vi "Set_up_controls.vi"(4 "error in":errorcluster, 5 "reference":refnum<vi>, 6 "FP refnum in":cluster{"server refnum":u32, "tag refnum":u32}, 7 "Data in":T1) -> (0 "error out":errorcluster, 1 "reference out":refnum<vi>, 2 "FP refnum out":cluster{"server refnum":u32, "tag refnum":u32}, 3 "Data out":T1)   [LabVIEW 2015, in "Steps.lvlib"]
uses:
  Steps.lvlib
  Type_Defs/Data.ctl
  Type_Defs/Diagnostics.ctl
  Type_Defs/Systems.ctl
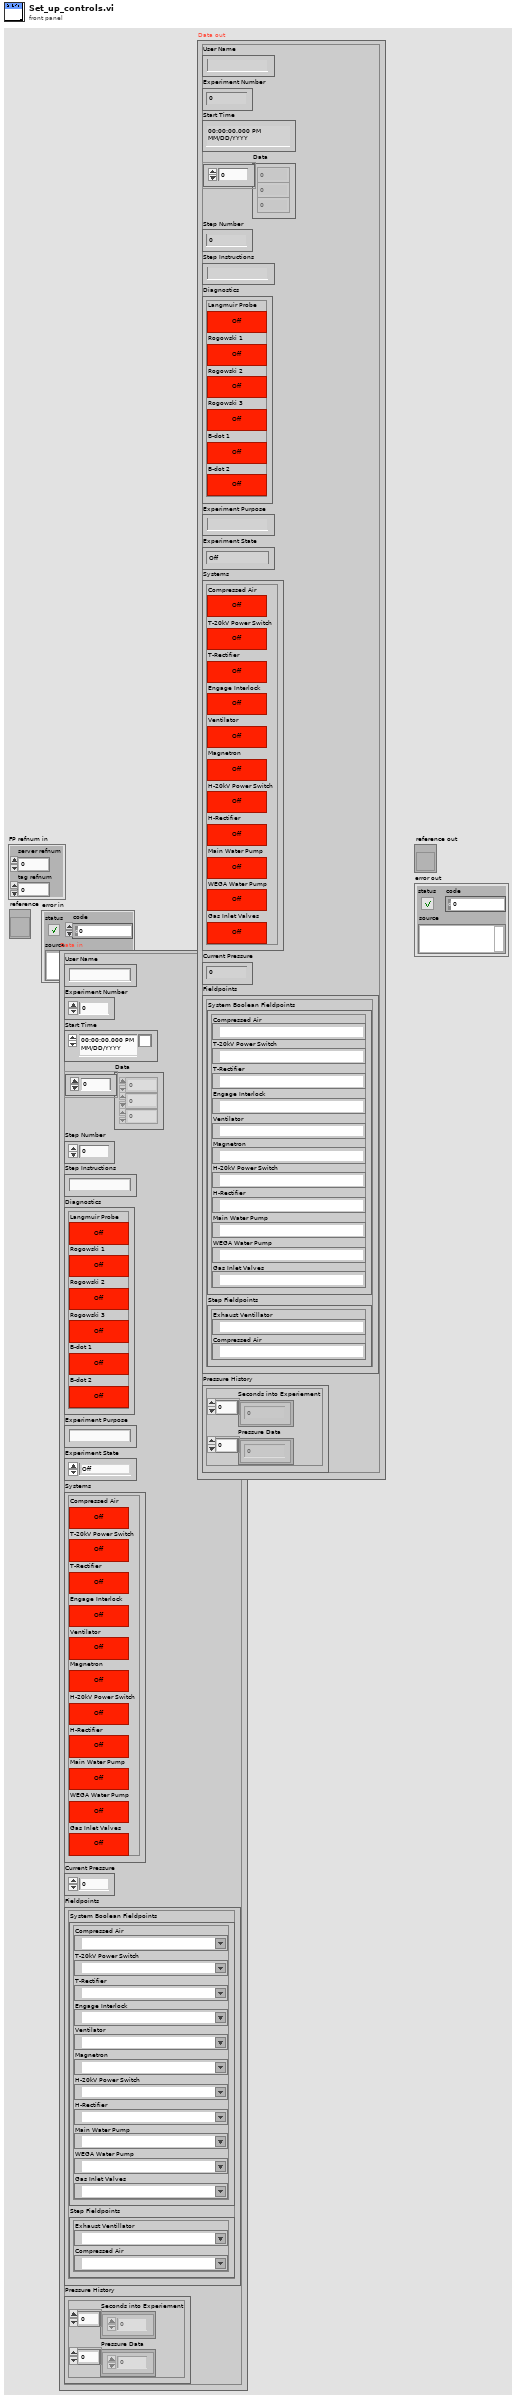
[diagram p1: front panel]
types:
  T1 = typedef "Data.ctl" = cluster{"User Name":string, "Experiment Number":i32, "Start Time":timestamp, "Data":dbl[], "Step Number":i32, "Step Instructions":string, "Diagnostics":T2, "Experiment Purpose":string, "Experiment State":enum16{"Off", "Setting Up", "Ready", "In Progress", "Shutting Down"}, "Systems":T3, "Current Pressure":dbl, "Fieldpoints":cluster{"System Boolean Fieldpoints":cluster{"Compressed Air":refnum<k21>, "T-20kV Power Switch":refnum<k21>, "T-Rectifier":refnum<k21>, "Engage Interlock":refnum<k21>, "Ventilator":refnum<k21>, "Magnetron":refnum<k21>, "H-20kV Power Switch":refnum<k21>, "H-Rectifier":refnum<k21>, "Main Water Pump":refnum<k21>, "WEGA Water Pump":refnum<k21>, "Gas Inlet Valves":refnum<k21>}, "Step Fieldpoints":cluster{"Exhaust Ventillator":refnum<k21>, "Compressed Air":refnum<k21>}}, "Pressure History":cluster{"Seconds into Experiement":i32[], "Pressure Data":dbl[]}}
  T2 = typedef "Diagnostics.ctl" = cluster{"Langmuir Probe":bool, "Rogowski 1":bool, "Rogowski 2":bool, "Rogowski 3":bool, "B-dot 1":bool, "B-dot 2":bool}
  T3 = typedef "Systems.ctl" = cluster{"Compressed Air":bool, "T-20kV Power Switch":bool, "T-Rectifier":bool, "Engage Interlock":bool, "Ventilator":bool, "Magnetron":bool, "H-20kV Power Switch":bool, "H-Rectifier":bool, "Main Water Pump":bool, "WEGA Water Pump":bool, "Gas Inlet Valves":bool}
  T4 = enum16{"Off", "Setting Up", "Ready", "In Progress", "Shutting Down"}
  T5 = enum8{"Enabled", "Disabled", "Disabled and Grayed Out"}
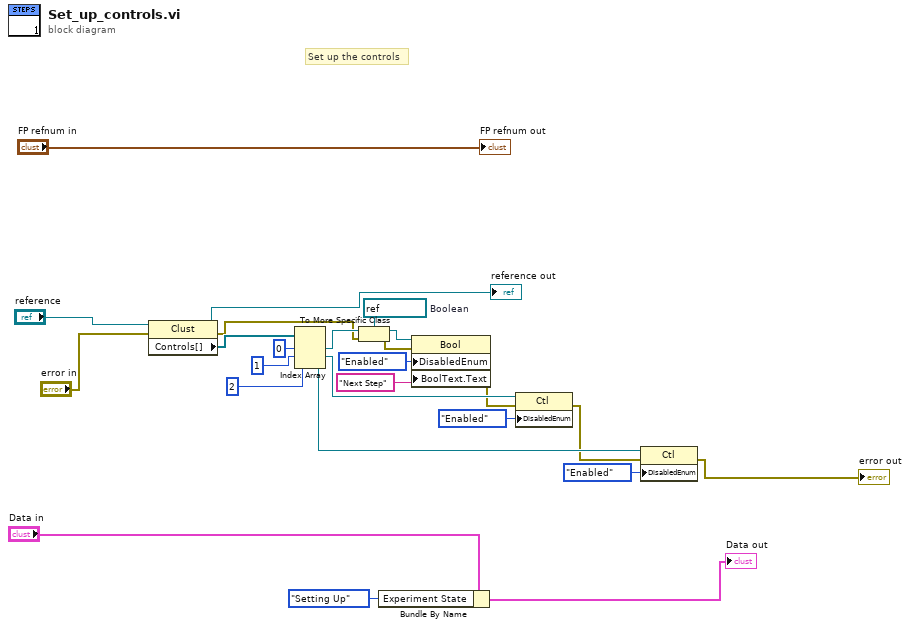
[diagram p0: block diagram]
diagram:
  w5 = refnum<vi> refnum  # Boolean
  # "Set up the controls"
  n1 = property class="Clust"(reference="reference", error in="error in") -> (reference out=→"reference out":refnum<vi>, error out=w8:errorcluster, "Controls[]"=w25:refnum<vi>[])
  n2 = Index Array(array=w25, index #1=0 ("index"), index #2=1 ("index"), index #3=2 ("index")) -> (element #1=w9:refnum<vi>, element #2=w21:refnum<vi>, element #3=w20:refnum<vi>)
  n3 = To More Specific Class(target class=w5, reference=w9, error in=w8) -> (specific class reference=w7:refnum<vi>, error out=w6:errorcluster)
  n4 = Bundle By Name(cluster="Data in", "Experiment State"=T4."Setting Up") -> (→"Data out":T1)
  n5 = property class="Bool"(reference=w7, error in=w6, "DisabledEnum"=T5."Enabled" ("Disabled"), "BoolText.Text"="Next Step" ("Boolean Text.Text")) -> (error out=w19:errorcluster)  [unwired: 1 out]
  n6 = property class="Ctl"(reference=w21, error in=w19, "DisabledEnum"=T5."Enabled" ("Disabled")) -> (error out=w18:errorcluster)  [unwired: 1 out]
  n7 = property class="Ctl"(reference=w20, error in=w18, "DisabledEnum"=T5."Enabled" ("Disabled")) -> (error out=→"error out":errorcluster)  [unwired: 1 out]
  "FP refnum out" <- "FP refnum in"
